vi "DutyCycles.vi"(2 "AnalogTriggers":T1[](array[typedef])=[{"InHysteresis"=FALSE, "OverLimit"=FALSE, "Rising"=FALSE, "Falling"=FALSE}, {"InHysteresis"=FALSE, "OverLimit"=FALSE, "Rising"=FALSE, "Falling"=FALSE}, {"InHysteresis"=FALSE, "OverLimit"=FALSE, "Rising"=FALSE, "Falling"=FALSE}, {"InHysteresis"=FALSE, "OverLimit"=FALSE, "Rising"=FALSE, "Falling"=FALSE}, {"InHysteresis"=FALSE, "OverLimit"=FALSE, "Rising"=FALSE, "Falling"=FALSE}, {"InHysteresis"=FALSE, "OverLimit"=FALSE, "Rising"=FALSE, "Falling"=FALSE}, {"InHysteresis"=FALSE, "OverLimit"=FALSE, "Rising"=FALSE, "Falling"=FALSE}, {"InHysteresis"=FALSE, "OverLimit"=FALSE, "Rising"=FALSE, "Falling"=FALSE}], 3 "DigitalInputs":bool[](array[boolean])=[FALSE, FALSE, FALSE, FALSE, FALSE, FALSE, FALSE, FALSE, FALSE, FALSE, FALSE, FALSE, FALSE, FALSE, FALSE, FALSE, FALSE, FALSE, FALSE, FALSE, FALSE, FALSE, FALSE, FALSE, FALSE, FALSE, FALSE, FALSE, FALSE, FALSE, FALSE, FALSE], 4 "Sources":T4) -> (0 "Frequencies":T2 {"DutyCycle7_Frequency" format="%.21g"; "DutyCycle6_Frequency" format="%.21g"; "DutyCycle5_Frequency" format="%.21g"; "DutyCycle4_Frequency" format="%.21g"; "DutyCycle3_Frequency" format="%.21g"; "DutyCycle2_Frequency" format="%.21g"; "DutyCycle1_Frequency" format="%.21g"; "DutyCycle0_Frequency" format="%.21g"}, 1 "Outputs":T3)   [LabVIEW 2019]
uses:
  Controls/DutyCycle_Sources.ctl
  Helpers/Source.ctl
  Controls/DutyCycle_Outputs.ctl
  Controls/DutyCycle_Frequencies.ctl
  Helpers/AnalogTriggerOutput.ctl
  <vilib>/rvi/Emulation/niFpgaSctlEmulationGetInTimedLoop.vi
  <vilib>/rvi/Emulation/niFpgaProcessEmulError.vi
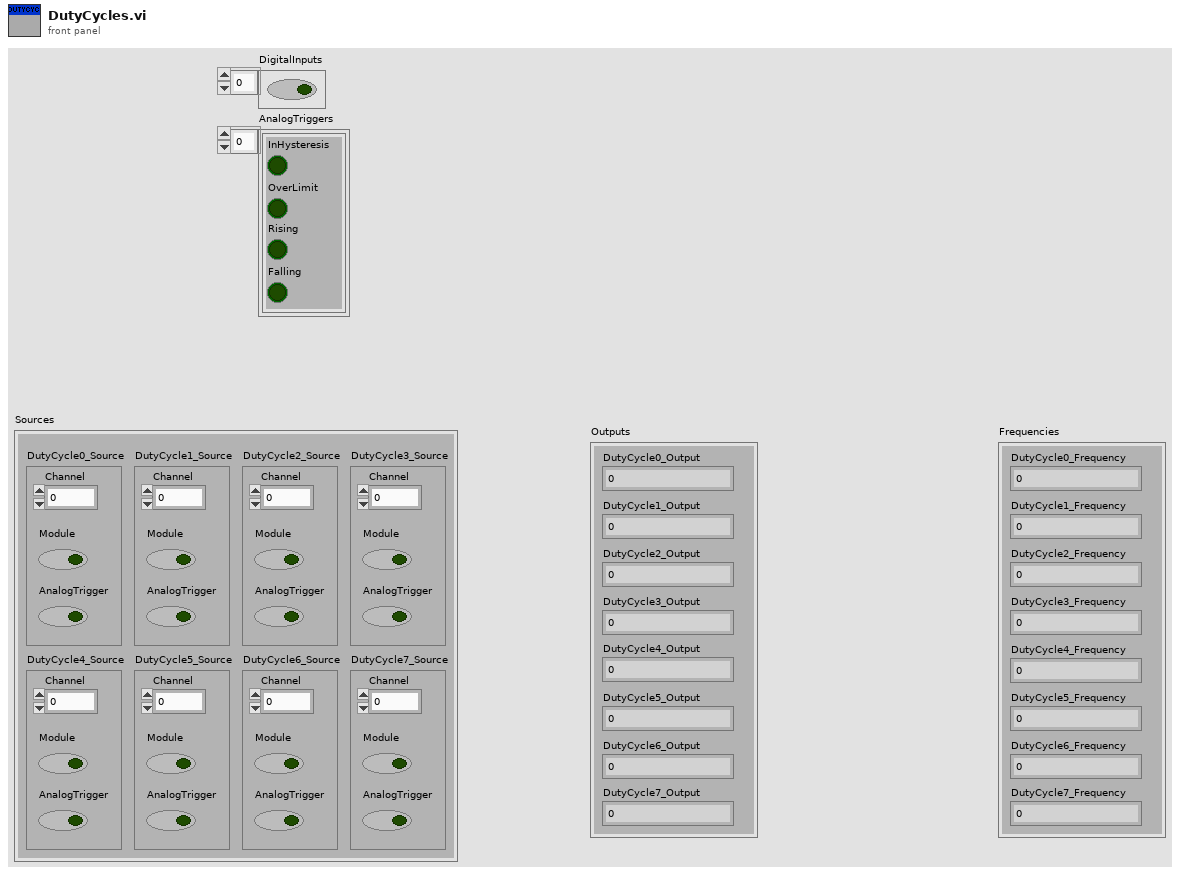
[diagram p1: front panel]
types:
  T1 = typedef "AnalogTriggerOutput.ctl" = cluster{"InHysteresis":bool, "OverLimit":bool, "Rising":bool, "Falling":bool}
  T2 = typedef "DutyCycle_Frequencies.ctl" = cluster{"DutyCycle0_Frequency":fxp<+,11,11>, "DutyCycle1_Frequency":fxp<+,11,11>, "DutyCycle2_Frequency":fxp<+,11,11>, "DutyCycle3_Frequency":fxp<+,11,11>, "DutyCycle4_Frequency":fxp<+,11,11>, "DutyCycle5_Frequency":fxp<+,11,11>, "DutyCycle6_Frequency":fxp<+,11,11>, "DutyCycle7_Frequency":fxp<+,11,11>}
  T3 = typedef "DutyCycle_Outputs.ctl" = cluster{"DutyCycle0_Output":fxp<+,31,31>, "DutyCycle1_Output":fxp<+,31,31>, "DutyCycle2_Output":fxp<+,31,31>, "DutyCycle3_Output":fxp<+,31,31>, "DutyCycle4_Output":fxp<+,31,31>, "DutyCycle5_Output":fxp<+,31,31>, "DutyCycle6_Output":fxp<+,31,31>, "DutyCycle7_Output":fxp<+,31,31>}
  T4 = typedef "DutyCycle_Sources.ctl" = cluster{"DutyCycle0_Source":T5, "DutyCycle1_Source":T5, "DutyCycle2_Source":T5, "DutyCycle3_Source":T5, "DutyCycle4_Source":T5, "DutyCycle5_Source":T5, "DutyCycle6_Source":T5, "DutyCycle7_Source":T5}
  T5 = typedef "Source.ctl" = cluster{"Channel":fxp<+,4,4>, "Module":bool, "AnalogTrigger":bool}
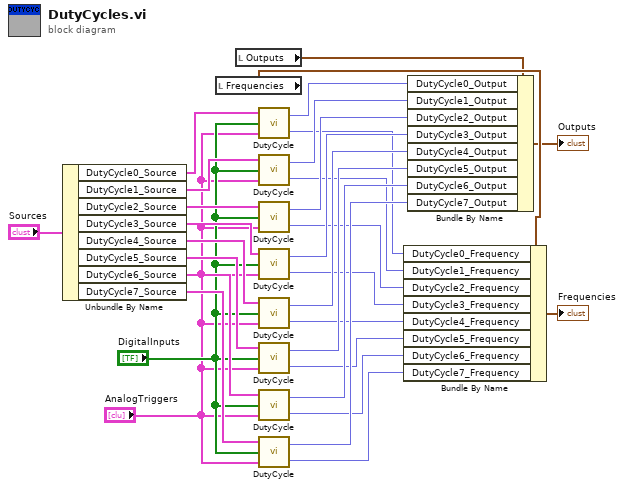
[diagram p0: block diagram]
diagram:
  n1 = Unbundle By Name("Sources") -> ("DutyCycle0_Source"=w26:T5, "DutyCycle1_Source"=w25:T5, "DutyCycle2_Source"=w24:T5, "DutyCycle3_Source"=w23:T5, "DutyCycle4_Source"=w22:T5, "DutyCycle5_Source"=w21:T5, "DutyCycle6_Source"=w20:T5, "DutyCycle7_Source"=w19:T5)
  n2 = local read "Frequencies"() -> (w30:T2)
  n3 = local read "Outputs"() -> (w28:T3)
  n4 = call "DutyCycle.vi"("AnalogTriggers"="AnalogTriggers", "DigitalInputs"="DigitalInputs", "Source"=w26) -> ("Frequency"=w10:fxp<+,11,11>, "Output"=w18:fxp<+,31,31>)
  n5 = call "DutyCycle.vi"("AnalogTriggers"="AnalogTriggers", "DigitalInputs"="DigitalInputs", "Source"=w25) -> ("Frequency"=w9:fxp<+,11,11>, "Output"=w17:fxp<+,31,31>)
  n6 = call "DutyCycle.vi"("AnalogTriggers"="AnalogTriggers", "DigitalInputs"="DigitalInputs", "Source"=w24) -> ("Frequency"=w8:fxp<+,11,11>, "Output"=w16:fxp<+,31,31>)
  n7 = call "DutyCycle.vi"("AnalogTriggers"="AnalogTriggers", "DigitalInputs"="DigitalInputs", "Source"=w23) -> ("Frequency"=w7:fxp<+,11,11>, "Output"=w15:fxp<+,31,31>)
  n8 = call "DutyCycle.vi"("AnalogTriggers"="AnalogTriggers", "DigitalInputs"="DigitalInputs", "Source"=w22) -> ("Frequency"=w6:fxp<+,11,11>, "Output"=w14:fxp<+,31,31>)
  n9 = call "DutyCycle.vi"("AnalogTriggers"="AnalogTriggers", "DigitalInputs"="DigitalInputs", "Source"=w21) -> ("Frequency"=w5:fxp<+,11,11>, "Output"=w13:fxp<+,31,31>)
  n10 = call "DutyCycle.vi"("AnalogTriggers"="AnalogTriggers", "DigitalInputs"="DigitalInputs", "Source"=w20) -> ("Frequency"=w4:fxp<+,11,11>, "Output"=w12:fxp<+,31,31>)
  n11 = call "DutyCycle.vi"("AnalogTriggers"="AnalogTriggers", "DigitalInputs"="DigitalInputs", "Source"=w19) -> ("Frequency"=w3:fxp<+,11,11>, "Output"=w11:fxp<+,31,31>)
  n12 = Bundle By Name(cluster=w30, "DutyCycle0_Frequency"=w10, "DutyCycle1_Frequency"=w9, "DutyCycle2_Frequency"=w8, "DutyCycle3_Frequency"=w7, "DutyCycle4_Frequency"=w6, "DutyCycle5_Frequency"=w5, "DutyCycle6_Frequency"=w4, "DutyCycle7_Frequency"=w3) -> (→"Frequencies":T2)
  n13 = Bundle By Name(cluster=w28, "DutyCycle0_Output"=w18, "DutyCycle1_Output"=w17, "DutyCycle2_Output"=w16, "DutyCycle3_Output"=w15, "DutyCycle4_Output"=w14, "DutyCycle5_Output"=w13, "DutyCycle6_Output"=w12, "DutyCycle7_Output"=w11) -> (→"Outputs":T3)
